vi "Image_Save_Dequeue.vi"(0 "Data":T1={"L16 Linear Actuator"="", "XE 1000 Pump"="", "Camera1"="", "Camera2"="", "Camera1_IMG"=refnum, "Camera2_IMG"=refnum, "Img_Capt"=FALSE, "Actuator"=FALSE, "Pump"=FALSE, "Cam 1"=FALSE, "Cam 2"=FALSE, "Empty_Refill"=FALSE, "Crop"=FALSE, "Light intensity"=100, "Exposure Time"=1000.0, "Sample Name"="Test Sample", "Operator"="MRJ", "Calibration 1"=path "C:/Users/au540322/Desktop/IHS_Project/images/Debris/Debris_0/Debris_0_2019_06_01-23-32-49-686.PNG", "Calibration 2"=path "C:/Users/au540322/Desktop/IHS_Project/images/Debris/Debris_0/Debris_0_2019_06_01-23-32-49-686.PNG", "Framerate"=1, "Timeout Sample"=0, "Collection date"="MRJ", "Sample size threshold"=1, "Empty start"=1, "Command"="MRJ", "Calibration Image 1"=refnum, "Calibration Image 2"=refnum, "Original Image 1"=refnum, "Original Image 2"=refnum, "Processing Image 1"=refnum, "Processing Image 2"=refnum, "Object Image 1"=refnum, "Object Image 2"=refnum, "Cam 1 - save queue"=refnum, "Cam 2 - save queue"=refnum, "Station"="", "Species Name"="", "Other Notes"="", "Aperture"=enum."Item 0", "Image Process Queue Size"=500, "Image Save Queue Size"=500, "Overload threshold"=500, "Max Framerate"=100, "Blue Plane Image"=refnum, "Subtract Image"=refnum, "Binary Image 1"=refnum, "ROI mask allocation"=refnum, "Rectangle 1"={"Left"=0, "Top"=0, "Right"=0, "Bottom"=0, "Rotation"=0.0}, "Rectangle 2"={"Left"=0, "Top"=0, "Right"=0, "Bottom"=0, "Rotation"=0.0}, "Binary Image 2"=refnum, "Detection Region %"=0.0, "Cam 1 queue"=refnum, "Cam 2 queue"=refnum, "Detect image 1"=refnum, "Detect image 2"=refnum, "Detect 1"=path "C:/Users/au540322/Desktop/IHS_Project/images/Debris/Debris_0/Debris_0_2019_06_01-23-32-49-686.PNG", "Detect 2"=path "C:/Users/au540322/Desktop/IHS_Project/images/Debris/Debris_0/Debris_0_2019_06_01-23-32-49-686.PNG", "Max large object threshold"=0, "Open(T)/Close(F)"=FALSE} {"Rectangle 2"."Rotation" format="%.2f"; "Rectangle 2"."Left" scale=0.0..1024.0; "Rectangle 2"."Right" scale=0.0..1024.0; "Rectangle 1"."Rotation" format="%.2f"; "Rectangle 1"."Left" scale=0.0..1024.0; "Rectangle 1"."Right" scale=0.0..1024.0; "Max Framerate" min=1; "Overload threshold" min=1; "Image Save Queue Size" min=1; "Image Process Queue Size" min=1; "Empty start" min=1; "Sample size threshold" min=1; "Framerate" min=1; "Light intensity" scale=0.0..100.0}, 5 "Camera":T5, 7 "Old":i32, 9 "Other":i32, 11 "Queue active":bool) -> (4 "# elements in queue":i32, 6 "State out":i32, 15 "Last image":bool)   [LabVIEW 2019]
uses:
  Camera_ID.ctl
  controls/Data.ctl
  <vilib>/userdefined/High Color/IMAQdx.ctl
  <vilib>/vision/Image Controls.llb/IMAQ Image.ctl
panel:
  out "error out":errorcluster
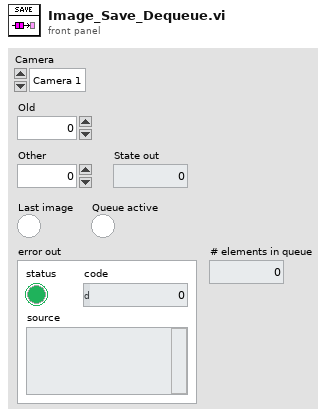
[diagram p1: front panel]
types:
  T1 = typedef "Data.ctl" = cluster{"L16 Linear Actuator":refnum<visa-resource-name>, "XE 1000 Pump":refnum<visa-resource-name>, "Camera1":T2, "Camera2":T2, "Camera1_IMG":T3, "Camera2_IMG":T3, "Img_Capt":bool, "Actuator":bool, "Pump":bool, "Cam 1":bool, "Cam 2":bool, "Empty_Refill":bool, "Crop":bool, "Light intensity":i32, "Exposure Time":dbl, "Sample Name":string, "Operator":string, "Calibration 1":path, "Calibration 2":path, "Framerate":i32, "Timeout Sample":i32, "Collection date":string, "Sample size threshold":i32, "Empty start":u32, "Command":string, "Calibration Image 1":T3, "Calibration Image 2":T3, "Original Image 1":T3, "Original Image 2":T3, "Processing Image 1":T3, "Processing Image 2":T3, "Object Image 1":T3, "Object Image 2":T3, "Cam 1 - save queue":refnum<queue>, "Cam 2 - save queue":refnum<queue>, "Station":string, "Species Name":string, "Other Notes":string, "Aperture":enum32{"Item 0", "Item 1", "Item 2", "Item 3"}, "Image Process Queue Size":i32, "Image Save Queue Size":i32, "Overload threshold":i32, "Max Framerate":i32, "Blue Plane Image":T3, "Subtract Image":T3, "Binary Image 1":T3, "ROI mask allocation":T3, "Rectangle 1":T4, "Rectangle 2":T4, "Binary Image 2":T3, "Detection Region %":dbl, "Cam 1 queue":refnum<queue>, "Cam 2 queue":refnum<queue>, "Detect image 1":T3, "Detect image 2":T3, "Detect 1":path, "Detect 2":path, "Max large object threshold":i32, "Open(T)/Close(F)":bool}
  T2 = typedef "IMAQdx.ctl" = refnum<k21>
  T3 = typedef "IMAQ Image.ctl" = refnum<image>
  T4 = typedef "IMAQ Rectangle" = cluster{"Left":i32, "Top":i32, "Right":i32, "Bottom":i32, "Rotation":dbl}
  T5 = typedef "Camera_ID.ctl" = enum16{"Camera 1", "Camera 2"}
  T6 = typedef "Image Type" = u32
  T7 = cluster{"Timestamp":string, "Image Pixels (U32)":u32[][], "Numeric":i32}
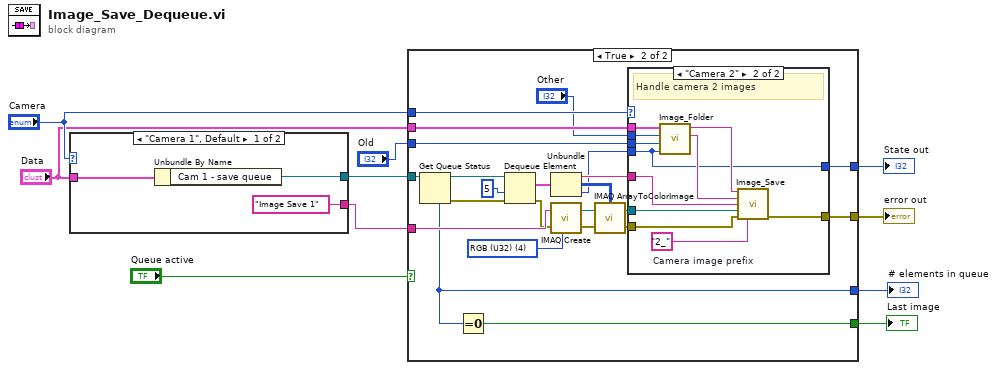
[diagram p0: block diagram]
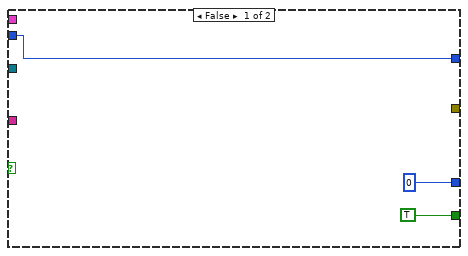
[diagram p2: hidden frame]
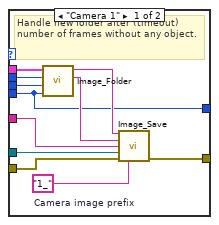
[diagram p3: hidden frame]
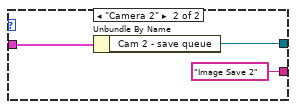
[diagram p4: hidden frame]
diagram:
  n1 = case shown="\"Camera 1\", Default" "Camera" {
    tunnel: [w12 w16] -> w8
    tunnel: "Data" -> [w13 w15]
    tunnel: ["Image Save 1" ("Image Name") "Image Save 2" ("Image Name")] -> w9
    frame "Camera 1", Default {
      n2 = Unbundle By Name(w13) -> ("Cam 1 - save queue"=w12:refnum<queue>)
    }
    frame "Camera 2" {
      n3 = Unbundle By Name(w15) -> ("Cam 2 - save queue"=w16:refnum<queue>)
    }
  }
  n4 = case shown="True" "Queue active" {
    tunnel: "Camera" -> [_ w42]
    tunnel: w9 -> [_ w38]
    tunnel: w8 -> [_ w33]
    tunnel: "Data" -> [_ w32]
    tunnel: [0 ("# elements in queue") w31] -> w5
    tunnel: [TRUE w30] -> w4
    tunnel: [_ w29] -> w3
    tunnel: [w17 w21] -> w2
    tunnel: "Old" -> [w17 w20]
    frame False {
    }
    frame True {
      w37 = T6 4 items=["Grayscale (U8)", "Grayscale (I16)", "Grayscale (SGL)", "Complex (CSG)", "RGB (U32)", "HSL (U32)", "RGB (U64)", "Grayscale (U16)"] ("Image Type")
      n5 = Get Queue Status(queue=w33) -> (queue out=w34:refnum<queue>, error out=w24:errorcluster, # elements in queue=w31:i32)  [unwired: 2 in, 5 out]
      n6 = Equal To 0?(x=w31) -> (x = 0?=w30:bool)
      n7 = Dequeue Element(queue=w34, timeout in ms (-1)=5, error in (no error)=w24) -> (element=w40:T7, error out=w25:errorcluster)  [unwired: 2 out]
      n8 = Unbundle(w40) -> ("Timestamp"=w28:string, "Image Pixels (U32)"=w39:u32[][], "Numeric"=w23:i32)
      n9 = call "IMAQ Create"("Image Name"=w38, "Image Type"=w37, "error in (no error)"=w25) -> ("New Image"=w36:T3, "error out"=w26:errorcluster)  [unwired: 2 in]
      n10 = call "IMAQ ArrayToColorImage"("Image Pixels (U32)"=w39, "Image"=w36, "error in (no error)"=w26) -> ("Image Out"=w35:T3, "error out"=w27:errorcluster)  [unwired: 2 in]
      n11 = case shown="\"Camera 2\"" w42 {
        tunnel: [w53 w64] -> w29
        tunnel: w35 -> [w52 w63]
        tunnel: w32 -> [w50 w61]
        tunnel: w28 -> [w47 w58]
        tunnel: w27 -> [w46 w57]
        tunnel: w23 -> [w43 w54]
        tunnel: w20 -> [w45 w56]
        tunnel: "Other" -> [w44 w55]
        tunnel: [w43 w54] -> w21
        frame "Camera 1" {
          w51 = "1_"  # Camera image prefix
          # "Handle new folder after (timeout) number of frames without any object."
          n12 = call "Image_Folder.vi"("New"=w43, "Old"=w45, "Other"=w44, "input cluster"=w50) -> ("Subfolder Name"=w48:string, "Subfolder Path"=w49:string)  [unwired: 6 in]
          n13 = call "Image_Save.vi"("Subfolder path"=w49, "Subfolder Name"=w48, "Timestamp"=w47, "Image in"=w52, "error in"=w46, "Camera"=w51) -> ("error out"=w53:errorcluster)  [unwired: 7 in, 2 out]
        }
        frame "Camera 2" {
          w62 = "2_"  # Camera image prefix
          # "Handle camera 2 images"
          n14 = call "Image_Folder.vi"("New"=w54, "Old"=w56, "Other"=w55, "input cluster"=w61) -> ("Subfolder Name"=w60:string, "Subfolder Path"=w59:string)  [unwired: 6 in]
          n15 = call "Image_Save.vi"("Subfolder path"=w59, "Subfolder Name"=w60, "Timestamp"=w58, "Image in"=w63, "error in"=w57, "Camera"=w62) -> ("error out"=w64:errorcluster)  [unwired: 7 in, 2 out]
        }
      }
    }
  }
  "# elements in queue" <- w5
  "Last image" <- w4
  "error out" <- w3
  "State out" <- w2
